vi "DAQ Thermocouple.vi"() -> ()   [LabVIEW 2019]
panel:
  in  "stop":bool
  out "Waveform Chart":dynamicdata(graph)
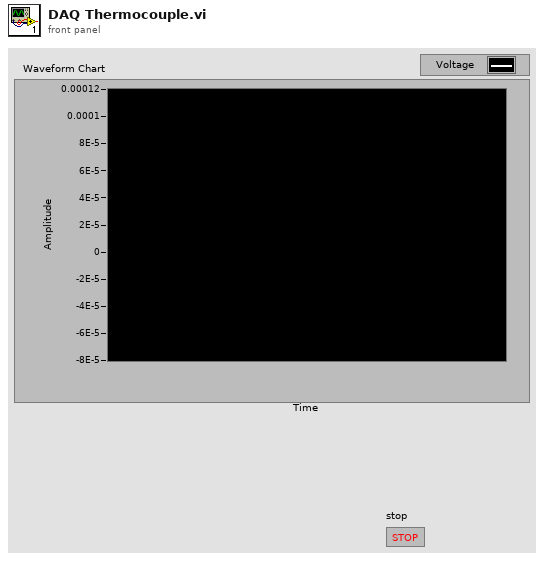
[diagram p1: front panel]
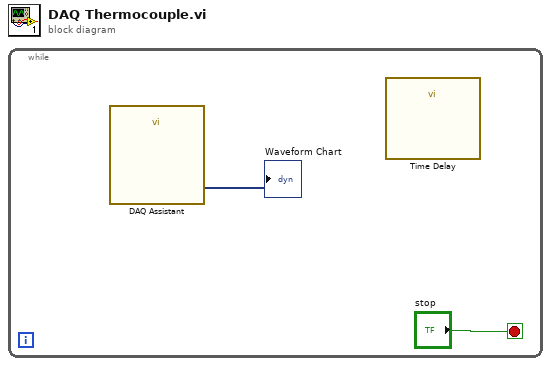
[diagram p0: block diagram]
diagram:
  n1 = while {
    stop <- "stop" stop-if-true
    n2 = call "DAQ Assistant"() -> ("data"=→"Waveform Chart":dynamicdata)  [unwired: 16 in, 3 out]
    n3 = call "Time Delay"() -> ()  [unwired: 11 in, 1 out]
  }
